vi "New Capture Cluster Constant.vi"(10 "Window ref angle":dbl, 11 "Bitfile name":string) -> (3 "Capture":T1)   [LabVIEW 2017, in "Engine Simulation Toolkit System Explorer.lvlib"]
uses:
  Engine Simulation Toolkit System Explorer.lvlib
  Event Timing Capture.ctl
  Event Reference Angle Selection.ctl
  Shared/Constants and GUIDs.vi
  Shared/Engine Simulation Toolkit Shared.lvlib
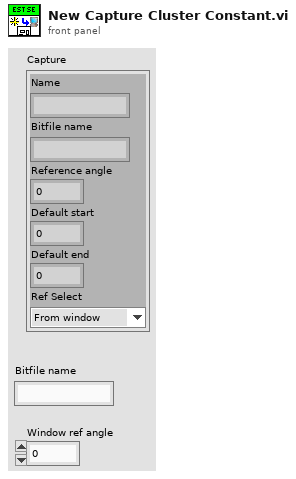
[diagram p1: front panel]
types:
  T1 = typedef "Engine Simulation Toolkit System Explorer.lvlib/Event Timing Capture.ctl" = cluster{"Name":string, "Bitfile name":string, "Reference angle":dbl, "Default start":dbl, "Default end":dbl, "Ref Select":T2}
  T2 = typedef "Engine Simulation Toolkit System Explorer.lvlib/Event Reference Angle Selection.ctl" = enum16{"From window", "Custom"}
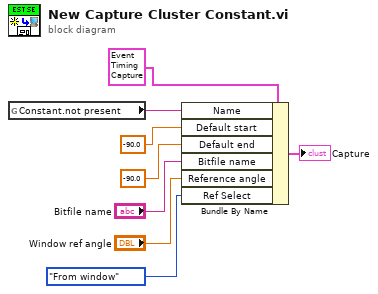
[diagram p0: block diagram]
diagram:
  n1 = global read "Constants and GUIDs.vi" "Constant.not present"() -> (w6:string)
  n2 = Bundle By Name(cluster=T1 {"Name"="", "Bitfile name"="", "Reference angle"=0.0, "Default start"=0.0, "Default end"=0.0, "Ref Select"=enum."From window"} ("Window"), "Name"=w6, "Default start"=-90.0, "Default end"=-90.0 ("Timeout"), "Bitfile name"="Bitfile name", "Reference angle"="Window ref angle", "Ref Select"=Event_Reference_Angle_Selection."From window") -> (→"Capture":T1)
